vi "Poly_WriteAnalogOut.vi"   [LabVIEW 2012]
doc: "Writes the specified \"Variable in\" value to the specified analog \"Channel\"."
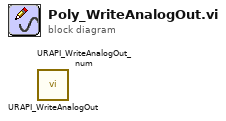
[diagram p0: block diagram]
diagram:
  n1 = call <userlib>:"URAPI_WriteAnalogOut.vi"() -> ()  [unwired: 4 in, 2 out]
  n2 = call <userlib>:"URAPI_WriteAnalogOut_num.vi"() -> ()  [unwired: 4 in, 2 out]
